vi "PWM.vi"(0 "Refnum in":refnum<k21>, 3 "High Time In 2":dbl, 5 "Speed 1":dbl, 6 "Speed 2/3":dbl, 7 "error in (no error)":errorcluster, 10 "High Time In 1":dbl) -> (20 "Refnum out":refnum<k21>, 22 "High Time Out 1":dbl, 23 "High Time Out 2":dbl, 27 "error out":errorcluster)   [LabVIEW 2011]
uses:
  <vilib>/DAQmx/write.llb/DAQmx Write (Counter 1D Time NChan 1Samp).vi
  <vilib>/DAQmx/miscellaneous.llb/DAQmx Fill In Error Info.vi
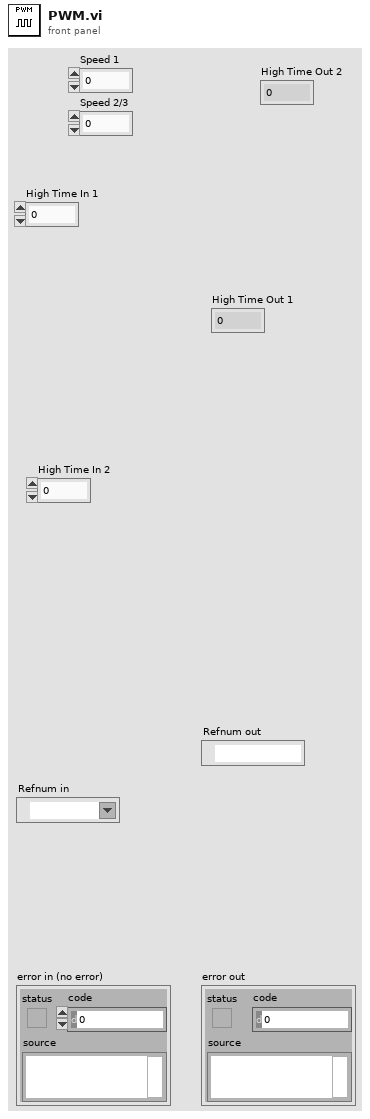
[diagram p1: front panel]
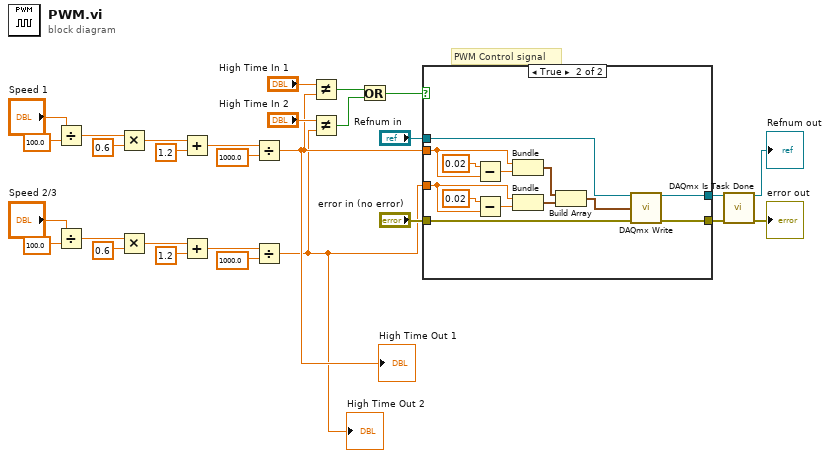
[diagram p0: block diagram]
diagram:
  # "PWM Control signal"
  n1 = Divide(x="Speed 1", y=100.0) -> (x/y=w20:dbl)
  n2 = Divide(x="Speed 2/3", y=100.0) -> (x/y=w13:dbl)
  n3 = Multiply(x=w20, y=0.6 ("scale")) -> (x*y=w22:dbl)
  n4 = Multiply(x=w13, y=0.6 ("scale")) -> (x*y=w15:dbl)
  n5 = Add(x=w22, y=1.2 ("add")) -> (x+y=w18:dbl)
  n6 = Add(x=w15, y=1.2 ("add")) -> (x+y=w11:dbl)
  n7 = Divide(x=w18, y=1000.0) -> (x/y=w4:dbl)
  "High Time Out 1" <- w4
  n8 = Divide(x=w11, y=1000.0) -> (x/y=w3:dbl)
  "High Time Out 2" <- w3
  n9 = Not Equal?(x="High Time In 1", y=w4) -> (x != y?=w8:bool)
  n10 = Not Equal?(x="High Time In 2", y=w3) -> (x != y?=w7:bool)
  n11 = Or(x=w8, y=w7) -> (x .or. y?=w23:bool)
  n12 = case shown="True" w23 {
    tunnel: [w31 w44] -> w27
    tunnel: [w30 w43] -> w28
    tunnel: "Refnum in" -> [w31 w42]
    tunnel: "error in (no error)" -> [w30 w41]
    tunnel: w3 -> [_ w36]
    tunnel: w4 -> [_ w32]
    frame False {
    }
    frame True {
      n13 = Subtract(x=0.02 ("total time"), y=w32) -> (x-y=w38:dbl)
      n14 = Subtract(x=0.02 ("total time"), y=w36) -> (x-y=w37:dbl)
      n15 = Bundle(w32, w38) -> (w35:cluster{dbl, dbl})  [unwired: 1 in]
      n16 = Bundle(w36, w37) -> (w34:cluster{dbl, dbl})  [unwired: 1 in]
      n17 = Build Array(w35, w34) -> (w33:cluster{dbl, dbl}[])
      n18 = call-poly <vilib>:"DAQmx Write.vi"("task/channels in"=w42, "data"=w33, "error in"=w41) -> ("task out"=w44:refnum<k21>, "error out"=w43:errorcluster)  [unwired: 10 in, 1 out]
    }
  }
  n19 = call <vilib>:"DAQmx Is Task Done.vi"("task/channels in"=w27, "error in"=w28) -> ("task out"=→"Refnum out":refnum<k21>, "error out"=→"error out":errorcluster)  [unwired: 11 in, 1 out]
